vi "GOMDBTS2048 is Measurement Quantity.vi"(8 "error in (no error)":errorcluster, 9 "quantity":string, 10 "calibrationEntryNumber":i32, 11 "handle":i32) -> (0 "error out":errorcluster, 1 "quantity out":string, 2 "function return":i32, 3 "isQuantity":bool)   [LabVIEW 2015, in "GOMDBTS2048.lvlib"]
doc: "GOBTS2048DLL int __stdcall GOMDBTS2048_isMeasurementQuantity(int handle, int calibrationEntryNumber, char *quantity, bool* isQuantity);"
uses:
  GOMDBTS2048.lvlib
  runtime/GOMDBTS2048.dll
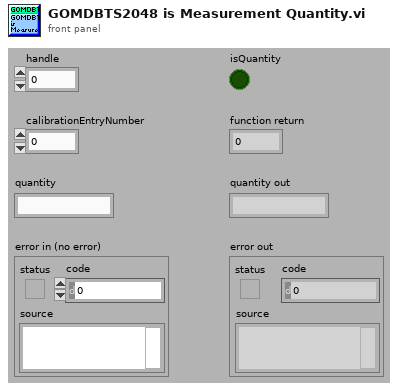
[diagram p1: front panel]
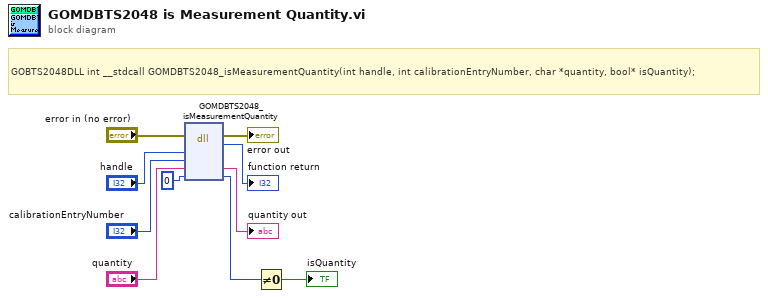
[diagram p0: block diagram]
diagram:
  # "GOBTS2048DLL int __stdcall GOMDBTS2048_isMeasurementQuantity(int handle, int calibrationEntryNumber, char *quantity, bool* isQuantity);"
  n1 = dll-call lib="C:/Users/rkoch/Documents/GO_Library/runtime/GOMDBTS2048.*" fn="GOMDBTS2048_isMeasurementQuantity"(error in="error in (no error)", "handle"="handle", "calibrationEntryNumber"="calibrationEntryNumber", "quantity"="quantity", "isQuantity"=u8 0) -> (error out=→"error out":errorcluster, →"function return":i32, "quantity"=→"quantity out":string, "isQuantity"=w3:u8)  [unwired: 4 in, 1 out]
  n2 = Not Equal To 0?(x=w3) -> (x != 0?=→"isQuantity":bool)
